vi "SP Find Filter Limit by Limit #.vi"(10 "Limit #":i8, 11 "Filter Limits":T1[](array[typedef]) {"Parameter"."Stimulus Port" min=1 step=1; "Parameter"."Response Port" min=1 step=1; "Passband"."Bandwidth Attn" format="%.3g"; "Passband"."Stop/Span" format="%.3g"; "Passband"."Start/Center" format="%.3g"}) -> (0 "Found?":bool, 3 "Filter Limit":T1={"Limit #"=1, "Parameter"={"Stimulus Port"=1, "Response Port"=2}, "Format"=enum."Log Mag", "Filter Type"=enum."Bandpass", "Passband"={"Start/Center"=500.0, "Stop/Span"=0.0, "Units"=enum."MHz", "Freq Format"=enum."Start/Stop", "Bandwidth Attn"=3.0, "Passband Limit"=FALSE}, "Ripple"={"Ripple Limit"=TRUE, "Window On"=FALSE, "Ripple"=0.1, "Window"=10.0, "Units"=enum."MHz"}, "Attenuation Points"=[], "Skirt Points"=[]} {"Parameter"."Stimulus Port" min=1 step=1; "Parameter"."Response Port" min=1 step=1; "Passband"."Bandwidth Attn" format="%.3g"; "Passband"."Stop/Span" format="%.3g"; "Passband"."Start/Center" format="%.3g"})   [LabVIEW 2011]
uses:
  TypeDefs/SP Filter.ctl
  TypeDefs/SP Parameter.ctl
  TypeDefs/SP Format.ctl
  TypeDefs/SP Filter Type.ctl
  TypeDefs/SP Filter Passband.ctl
  TypeDefs/SP Frequency Units.ctl
  TypeDefs/SP Frequency Format.ctl
  TypeDefs/SP Filter Ripple.ctl
  TypeDefs/SP Attenuation Point.ctl
  TypeDefs/SP Attenuation Type.ctl
  TypeDefs/SP Skirt Rejection Point.ctl
  TypeDefs/SP Relative Loss.ctl
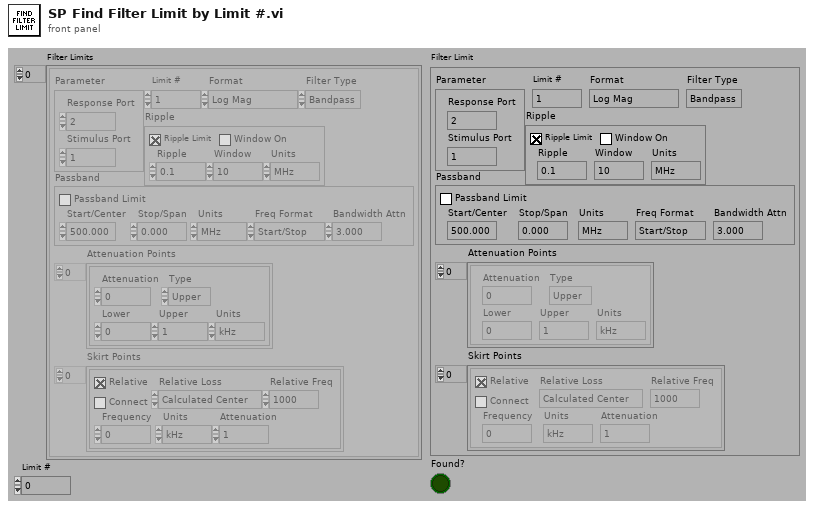
[diagram p1: front panel]
types:
  T1 = typedef "SP Filter.ctl" = cluster{"Limit #":i8, "Parameter":T2, "Format":T3, "Filter Type":T4, "Passband":T5, "Ripple":T8, "Attenuation Points":T9[], "Skirt Points":T11[]}
  T2 = typedef "SP Parameter.ctl" = cluster{"Stimulus Port":i8, "Response Port":i8}
  T3 = typedef "SP Format.ctl" = enum16{"Log Mag", "Lin Mag", "SWR", "Phase", "Expanded Phase", "Delay", "Insertion Loss", "Isolation", "Return Loss"}
  T4 = typedef "SP Filter Type.ctl" = enum16{"Lowpass", "Highpass", "Bandpass", "Bandstop"}
  T5 = typedef "SP Filter Passband.ctl" = cluster{"Start/Center":dbl, "Stop/Span":dbl, "Units":T6, "Freq Format":T7, "Bandwidth Attn":dbl, "Passband Limit":bool}
  T6 = typedef "SP Frequency Units.ctl" = enum16{"Hz", "kHz", "MHz", "GHz", "Points"}
  T7 = typedef "SP Frequency Format.ctl" = enum16{"Start/Stop", "Center/Span"}
  T8 = typedef "SP Filter Ripple.ctl" = cluster{"Ripple Limit":bool, "Window On":bool, "Ripple":dbl, "Window":dbl, "Units":T6}
  T9 = typedef "SP Attenuation Point.ctl" = cluster{"Attenuation":dbl, "Type":T10, "Lower":dbl, "Upper":dbl, "Units":T6}
  T10 = typedef "SP Attenuation Type.ctl" = enum16{"Center", "Lower", "Upper"}
  T11 = typedef "SP Skirt Rejection Point.ctl" = cluster{"Relative":bool, "Connect":bool, "Frequency":dbl, "Units":T6, "Attenuation":dbl, "Relative Loss":T12, "Relative Freq":dbl}
  T12 = typedef "SP Relative Loss.ctl" = enum16{"Calculated Center", "Passband Minimum", "Passband Maximum", "Passband Average", "Frequency"}
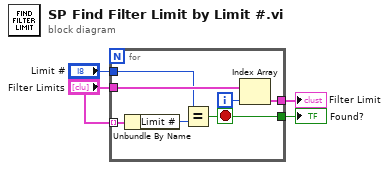
[diagram p0: block diagram]
diagram:
  n1 = for {
    tunnel: "Filter Limits" -> [w11] mode=indexing
    tunnel: "Filter Limits" -> [w10]
    tunnel: "Limit #" -> [w7]
    tunnel: [w6] -> w2
    tunnel: [w5] -> w1
    i -> [w9]
    stop <- w6 stop-if-true
    n2 = Unbundle By Name(w11) -> ("Limit #"=w8:i8)
    n3 = Equal?(x=w7, y=w8) -> (x = y?=w6:bool)
    n4 = Index Array(array=w10, index=w9) -> (element=w5:T1)
  }
  "Filter Limit" <- w1
  "Found?" <- w2
